vi "Launch.vi"() -> ()   [LabVIEW 2021, in "CIFCorePluginBuild.lvlib"]
uses:
  CIFCorePluginBuild.lvlib
  CIFCorePlugin.lvclass
  CIFCorePlugin.lvclass/CIFCorePlugin.ctl
  CIFUtilities/CIFLogs/CIFLogs.lvlib
panel:
  out "gRPC Server Port":i32
  in  "Plugin Name":string="Plugin Name Here"
  in  "host ip":string="localhost"
  in  "port":u16=1256
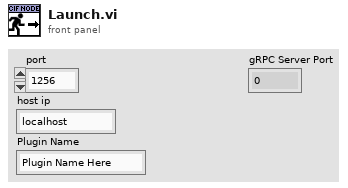
[diagram p1: front panel]
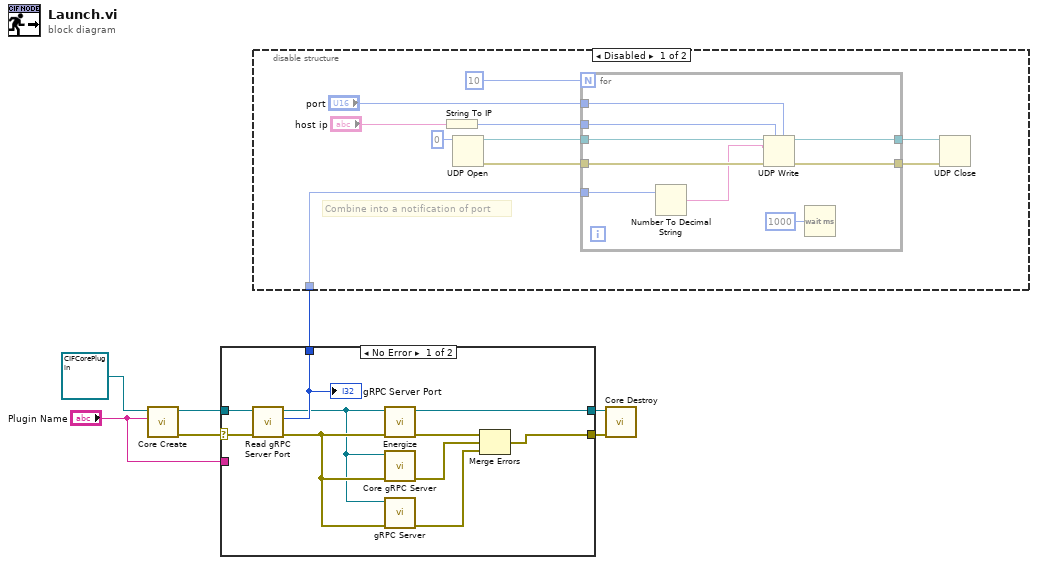
[diagram p0: block diagram]
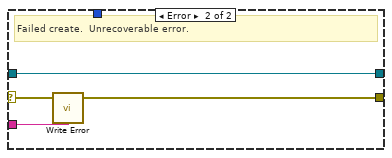
[diagram p3: hidden frame]
diagram:
  n1 = call "Core Create.vi"("Plugin Name"="Plugin Name", "CIFTemplateNode in"=refnum<class "CIFCorePlugin.lvclass"> refnum ("CIFCorePlugin.lvclass")) -> ("error out"=w2:errorcluster, "CIFTemplateNode out"=w5:refnum<class "CIFCorePlugin.lvclass">)  [unwired: 8 in]
  n2 = case shown="No Error" w2 {
    selector: w2 -> [w8 w21]
    tunnel: [w17 _] -> w7
    tunnel: [w16 w18] -> w6
    tunnel: w5 -> [w14 w18]
    tunnel: [w10 w19] -> w4
    tunnel: "Plugin Name" -> [_ w20]
    frame No Error {
      n3 = call "Read gRPC Server Port.vi"("error in (no error)"=w8, "CIFTemplateNode in"=w14) -> ("error out"=w15:errorcluster, "gRPC Server Port"=w17:i32, "CIFTemplateNode out"=w9:refnum<class "CIFCorePlugin.lvclass">)  [unwired: 7 in]
      "gRPC Server Port" <- w17
      n4 = call "Energize.vi"("error in (no error)"=w15, "CIFCorePlugin in"=w9) -> ("error out"=w13:errorcluster, "CIFCorePlugin out"=w16:refnum<class "CIFCorePlugin.lvclass">)  [unwired: 8 in]
      n5 = call "Core gRPC Server.vi"("error in (no error)"=w15, "CIFTemplateNode in"=w9) -> ("error out"=w12:errorcluster)  [unwired: 8 in, 1 out]
      n6 = call-dynamic "gRPC Server.vi"("error in (no error)"=w15, "CIFTemplateNode in"=w9) -> ("error out"=w11:errorcluster)  [unwired: 8 in, 1 out]
      n7 = Merge Errors(w13, w12, w11) -> (w10:errorcluster)
    }
    frame Error {
      # "Failed create.  Unrecoverable error."
      n8 = call "Write Error.vi"("error in (no error)"=w21, "Plugin Name"=w20) -> ("cleared error"=w19:errorcluster)  [unwired: 2 in]
    }
  }
  n9 = disable-structure shown="Disabled" {
    disable-tunnel: w7 -> [w31 _]
    frame Disabled {
      # "Combine into a notification of port"
      n10 = String To IP(1:"host ip") -> (0:w26:u32)
      n11 = UDP Open(11:u16 0 ("port")) -> (port=w29:refnum<k16>, 0:w28:errorcluster)  [unwired: 4 in, 1 out]
      n12 = for {
        N: 10 -> [_]
        tunnel: w29 -> [w40]
        tunnel: w28 -> [w39]
        tunnel: "port" -> [w38]
        tunnel: w26 -> [w37]
        tunnel: [w34] -> w23
        tunnel: [w33] -> w22
        tunnel: w31 -> [w32]
        n13 = Number To Decimal String(number=w32) -> (decimal integer string=w35:string)  [unwired: 1 in]
        n14 = UDP Write(address=w37, port or service name=w38, connection ID=w40, data in=w35, 8:w39) -> (error out=w33:errorcluster, 3:w34:refnum<k16>)  [unwired: 1 in]
        n15 = Wait (ms)(milliseconds to wait=u32 1000) -> ()  [unwired: 1 out]
      }
      n16 = UDP Close(connection ID=w23, 8:w22) -> ()  [unwired: 2 out]
    }
    frame Enabled {
    }
  }
  n17 = call "Core Destroy.vi"("error in (no error)"=w4, "CIFTemplateNode in"=w6) -> ()  [unwired: 8 in, 2 out]
